vi "CheckIfTDMS.vi"(6 "Label header with scale information (on/ OFF)":bool, 7 "View TDMS Header information (on/ off)":bool, 8 "error in (no error)":errorcluster, 9 "channel name":string="iq", 10 "Scale Data":dbl, 11 "original binary file Location":path) -> (0 "error out":errorcluster, 3 "Converted Binary to TDMS location":path)   [LabVIEW 2017]
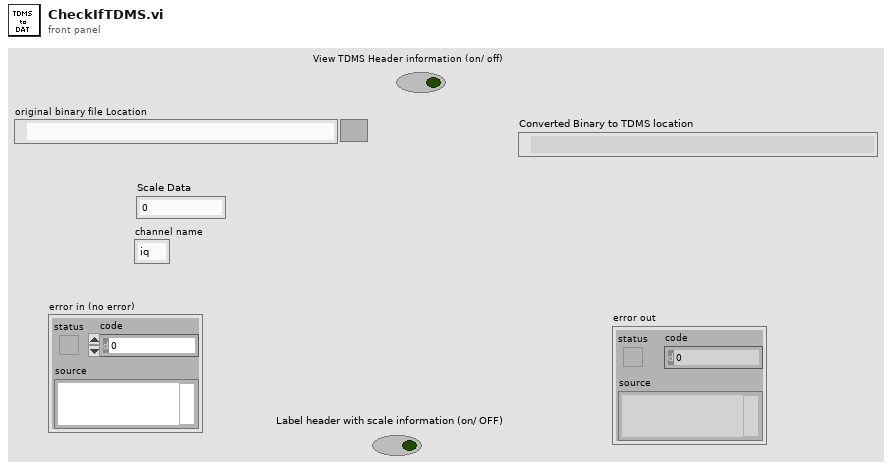
[diagram p1: front panel]
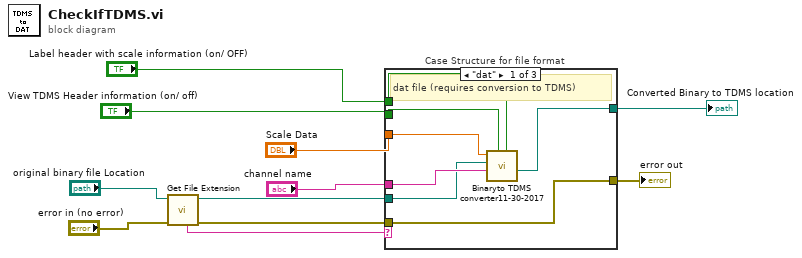
[diagram p0: block diagram]
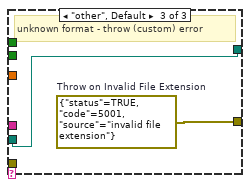
[diagram p3: hidden frame]
diagram:
  n1 = call <vilib>:"Get File Extension.vi"("error in (no error)"="error in (no error)", "file"="original binary file Location") -> ("error out"=w9:errorcluster, "dup file"=w6:path, "unmodified file extension"=w10:string)  [unwired: 5 in, 2 out]
  n2 = case "Case Structure for file format" shown="\"dat\"" w10 {
    tunnel: w9 -> [w18 w20 _]
    tunnel: [w18 w20 w21] -> w8
    tunnel: w6 -> [w12 w19 w22]
    tunnel: "channel name" -> [w13 _ _]
    tunnel: "Scale Data" -> [w16 _ _]
    tunnel: "View TDMS Header information (on/ off)" -> [w15 _ _]
    tunnel: "Label header with scale information (on/ OFF)" -> [w14 _ _]
    tunnel: [w17 w19 w22] -> w1
    frame "dat" {
      # "dat file (requires conversion to TDMS)"
      n3 = call "Binaryto TDMS converter11-30-2017.vi"("Label header with scale information (on/ OFF)"=w14, "View TDMS Header information (on/ off)"=w15, "channel name"=w13, "original binary file Location"=w12, "Scale Data"=w16) -> ("Converted Binary to TDMS location"=w17:path)  [unwired: 4 in, 2 out]
    }
    frame "tdms" {
      # "tdms file (is already in desired format)"
    }
    frame "other", Default {
      w21 = errorcluster {"status"=TRUE, "code"=5001, "source"="invalid file extension"}  # Throw on Invalid File Extension
      # "unknown format - throw (custom) error"
    }
  }
  "error out" <- w8
  "Converted Binary to TDMS location" <- w1
